vi "DevicesManager.vi"(8 "error in (no error)":errorcluster, 10 "Notifiers":T1, 11 "All Message Queue Cluster":T2) -> (0 "error out":errorcluster)   [LabVIEW 2017]
doc: "Ce VI a pour but de géré la connection des différents appareils.\n- Il permet de les connecté en fonction de leur port.\n- Il indique s'il se sont bien connecter et si tout se passe bien."
uses:
  Lib QMH/AllMessageQueue Cluster.ctl
  Lib QMH/Message Cluster.ctl
  Lib Notifier/Notifier.ctl
  Manager UI Data.ctl
  Lib QMH/MessageQueues.lvlib
  Lib Notifier/Notifier.lvlib
panel:
  in  "Portnumber Laser":i32(ring)=24 items=["COM1", "COM2", "COM3", "COM4", "COM5", "COM6", "COM7", "COM8", "COM9", "COM10", "COM11", "COM12", "COM13", "COM14", "COM15", "COM16", "COM17", "COM18", "COM19", "COM20", "COM21", "COM22", "COM23", "COM24", "COM25", "COM26", "COM27", "COM28", "COM29", "COM30"]
  out "Laser Initialized":bool
  out "Status Laser":string
  in  "Connect Laser":bool
  in  "Port Number Slit":i32(ring)=2 items=["COM1", "COM2", "COM3", "COM4", "COM5", "COM6", "COM7", "COM8", "COM9", "COM10", "COM11", "COM12", "COM13", "COM14", "COM15", "COM16", "COM17", "COM18", "COM19", "COM20", "COM21", "COM22", "COM23", "COM24", "COM25", "COM26", "COM27", "COM28", "COM29", "COM30"]
  in  "Portnumber Positioner":i32(ring)=17 items=["COM1", "COM2", "COM3", "COM4", "COM5", "COM6", "COM7", "COM8", "COM9", "COM10", "COM11", "COM12", "COM13", "COM14", "COM15", "COM16", "COM17", "COM18", "COM19", "COM20", "COM21", "COM22", "COM23", "COM24", "COM25", "COM26", "COM27", "COM28", "COM29", "COM30"]
  out "Positioner Initialized":bool
  out "Spectro Initialized":bool
  out "Slit Initialized":bool
  out "Status Spectro":string
  out "Status Slit":string
  out "Status Positioner":string
  in  "Connect Positioner":bool
  in  "Connect Slit":bool
  in  "Connect Spectro":bool
  # "Spectrometer"
  # "Slit"
  # "Selector"
  # "Laser"
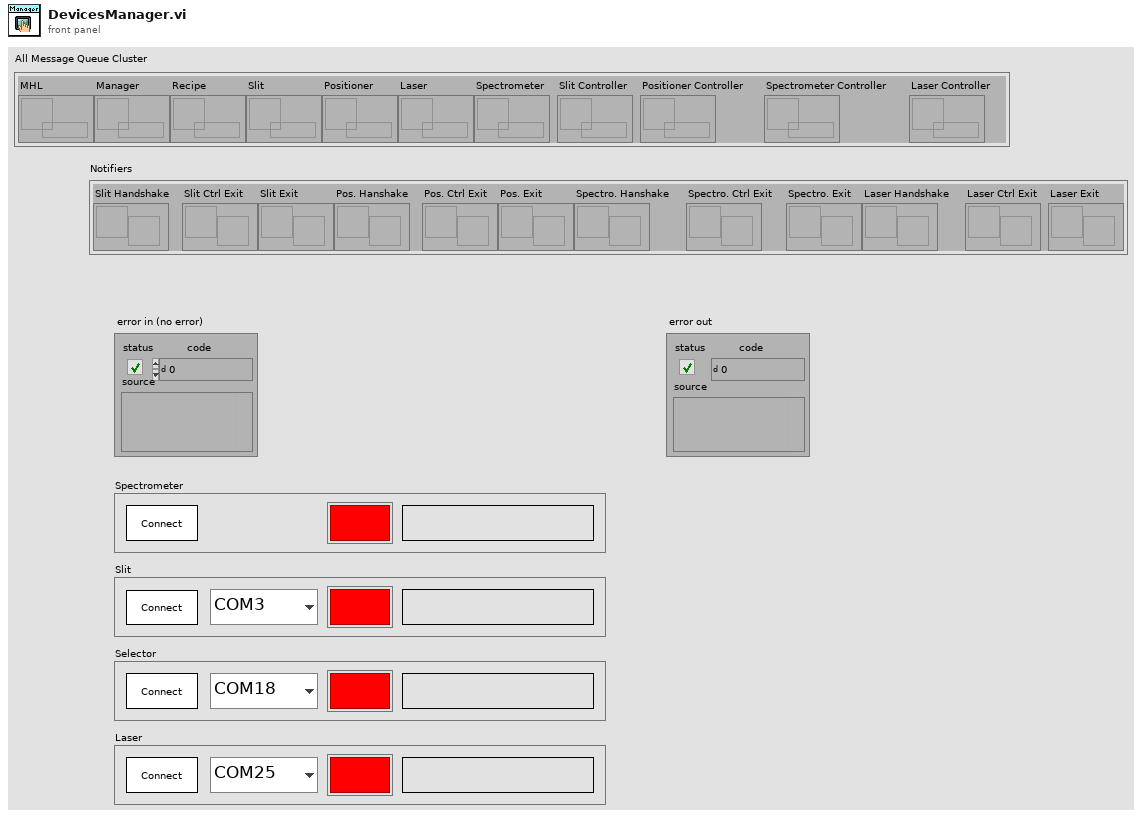
[diagram p1: front panel]
types:
  T1 = typedef "Notifier.lvlib/Notifier.ctl" = cluster{"Slit Handshake":refnum<notifier>, "Slit Ctrl Exit":refnum<notifier>, "Slit Exit":refnum<notifier>, "Pos. Hanshake":refnum<notifier>, "Pos. Ctrl Exit":refnum<notifier>, "Pos. Exit":refnum<notifier>, "Spectro. Hanshake":refnum<notifier>, "Spectro. Ctrl Exit":refnum<notifier>, "Spectro. Exit":refnum<notifier>, "Laser Handshake":refnum<notifier>, "Laser Ctrl Exit":refnum<notifier>, "Laser Exit":refnum<notifier>}
  T2 = typedef "MessageQueues.lvlib/AllMessageQueue Cluster.ctl" = cluster{"MHL":refnum<queue>, "Manager":refnum<queue>, "Recipe":refnum<queue>, "Slit":refnum<queue>, "Positioner":refnum<queue>, "Laser":refnum<queue>, "Spectrometer":refnum<queue>, "Slit Controller":refnum<queue>, "Positioner Controller":refnum<queue>, "Spectrometer Controller":refnum<queue>, "Laser Controller":refnum<queue>}
  T3 = typedef "Manager UI Data.ctl" = cluster{"Spectro Initialized":bool, "Status Spectro":string, "Slit Initialized":bool, "Status Slit":string, "Positioner Initialized":bool, "Status Positioner":string, "Laser Initialized":bool, "Status Laser":string}
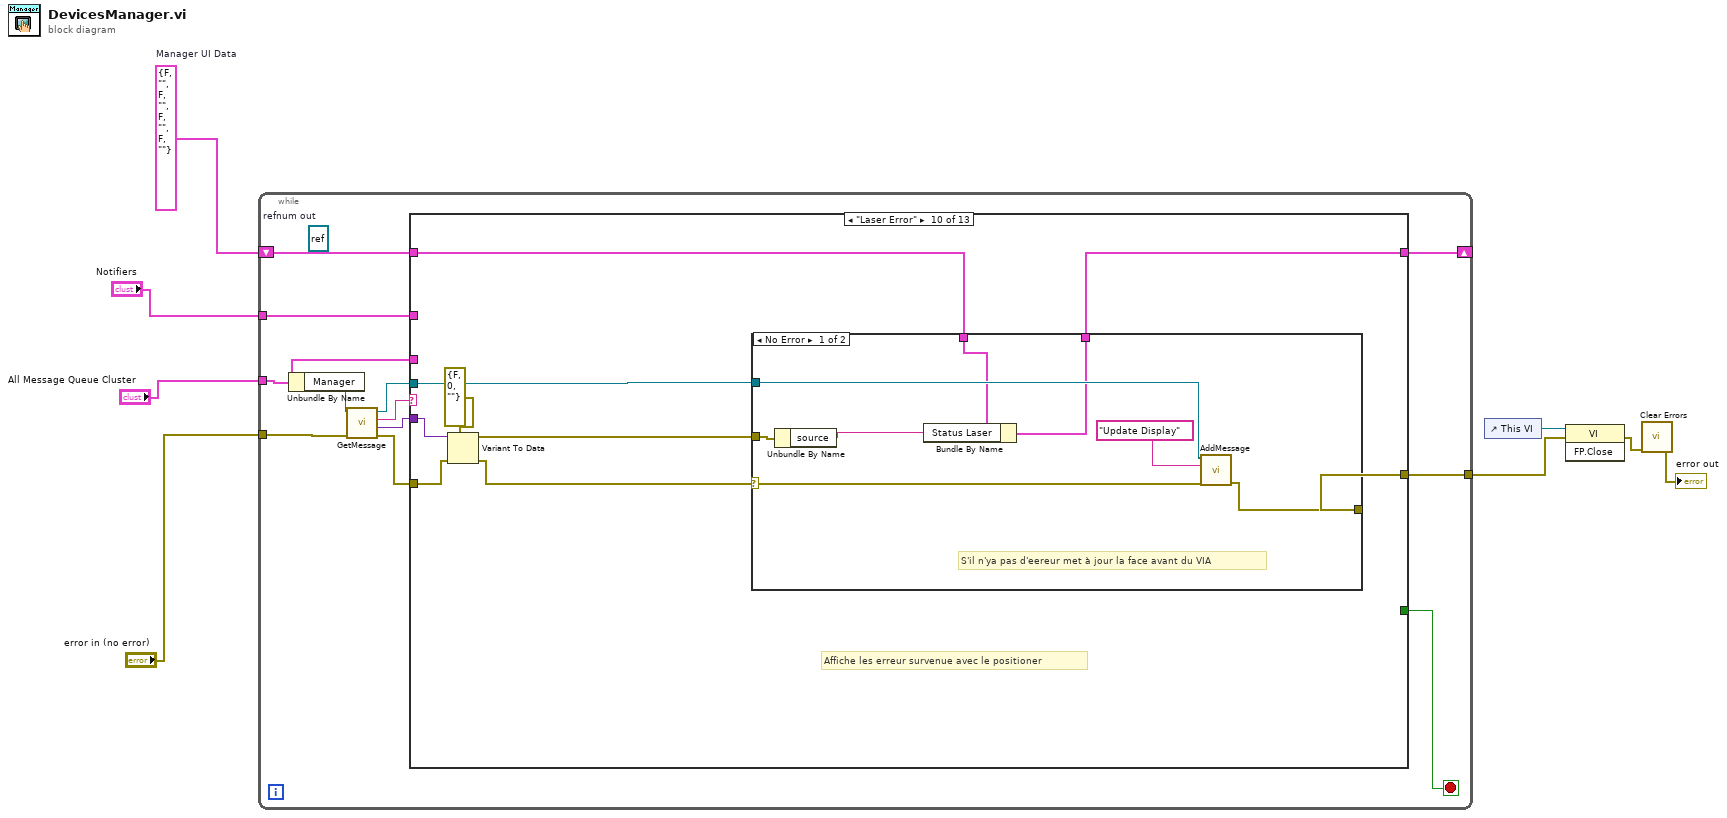
[diagram p0: block diagram]
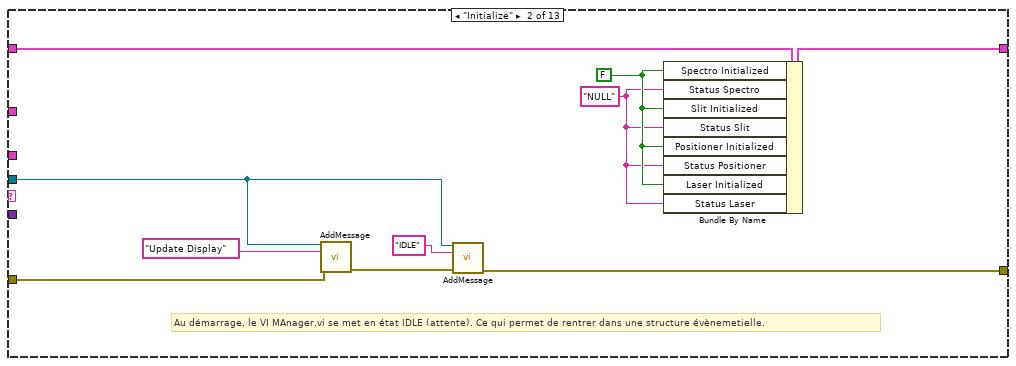
[diagram p3: hidden frame]
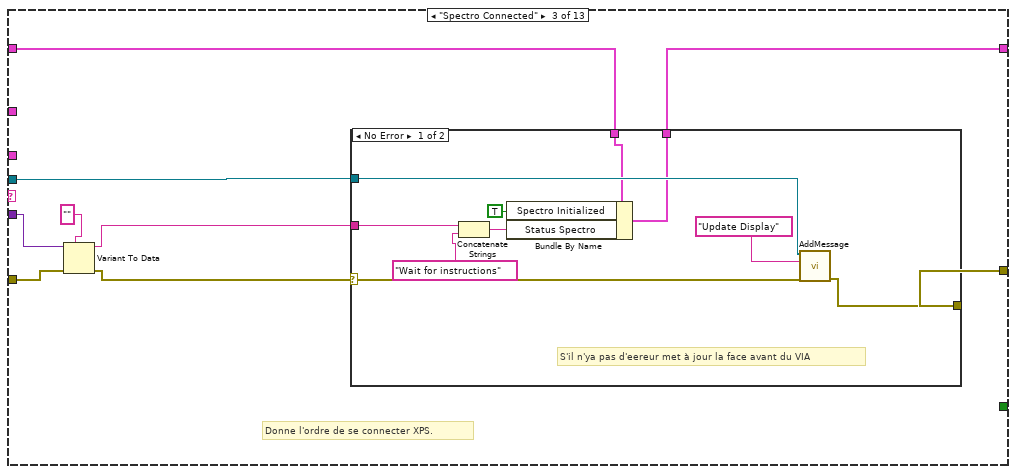
[diagram p4: hidden frame]
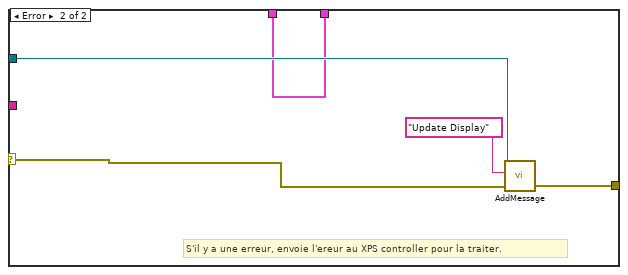
[diagram p5: hidden frame]
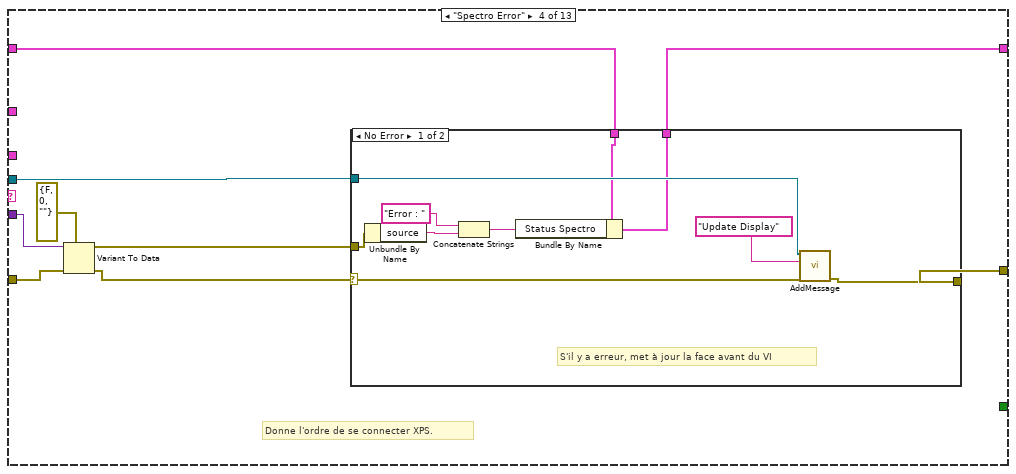
[diagram p6: hidden frame]
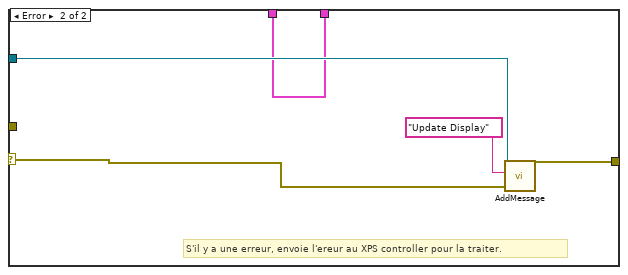
[diagram p7: hidden frame]
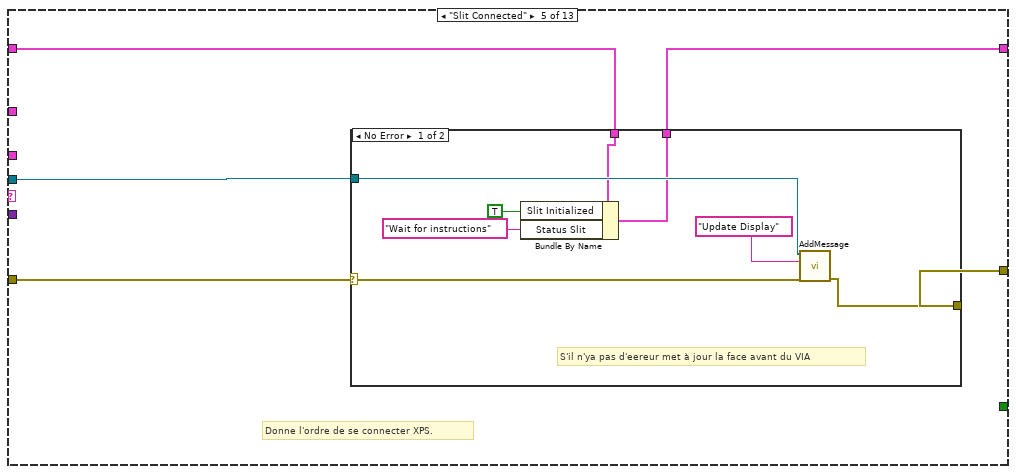
[diagram p8: hidden frame]
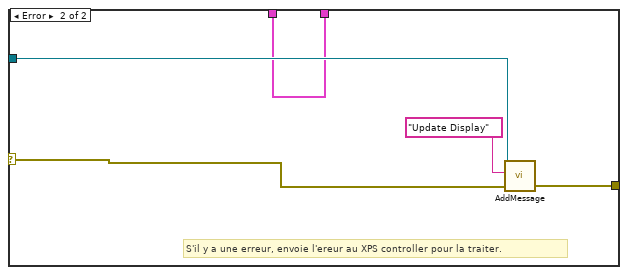
[diagram p9: hidden frame]
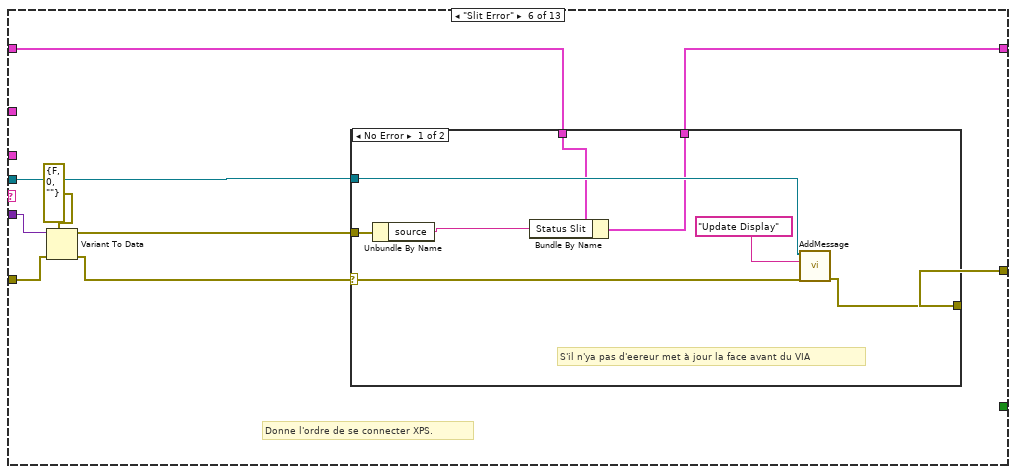
[diagram p10: hidden frame]
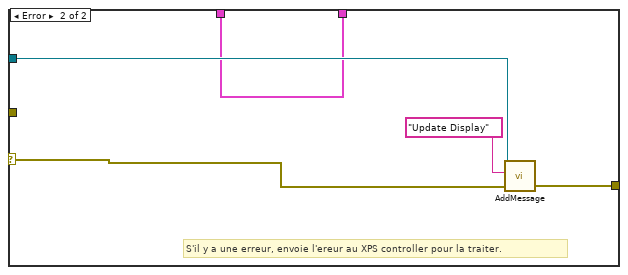
[diagram p11: hidden frame]
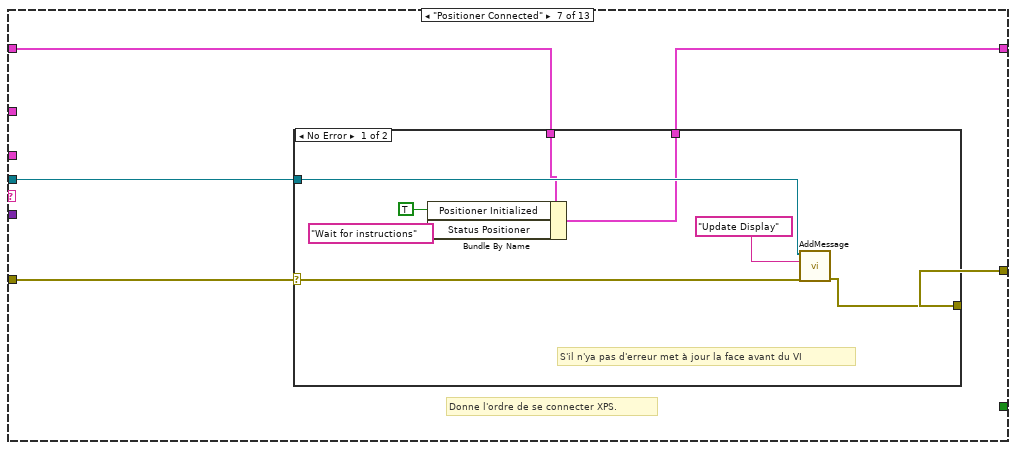
[diagram p12: hidden frame]
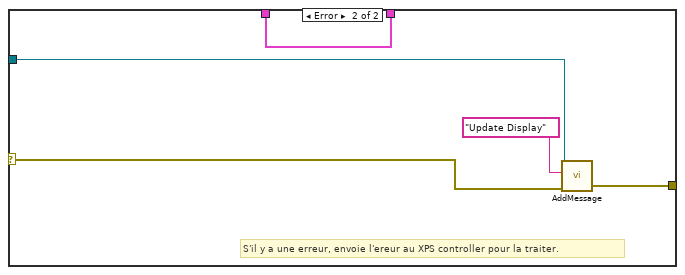
[diagram p13: hidden frame]
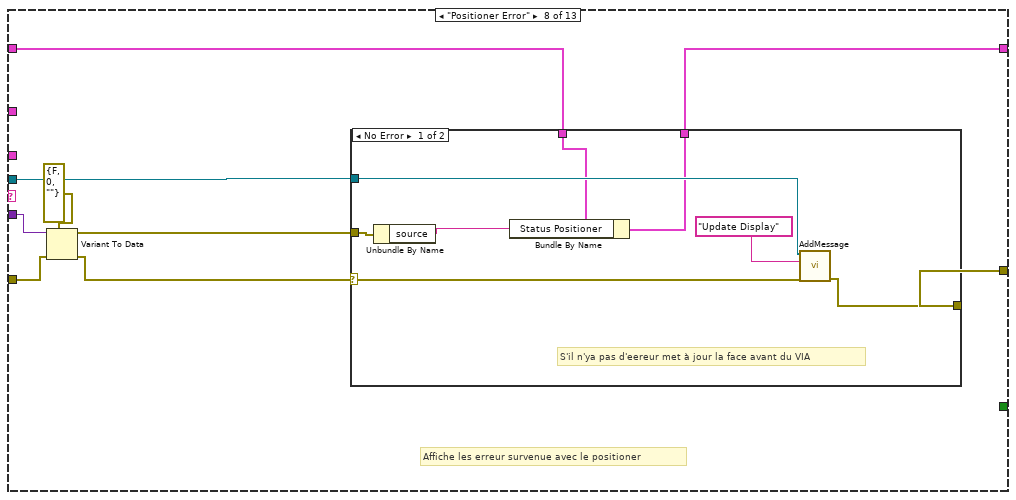
[diagram p14: hidden frame]
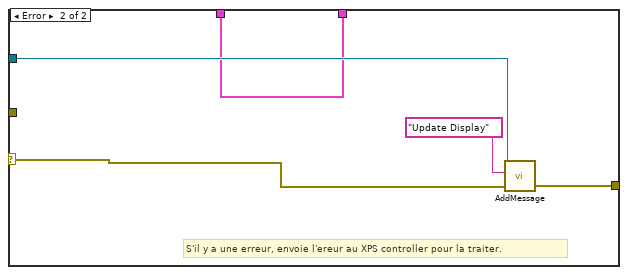
[diagram p15: hidden frame]
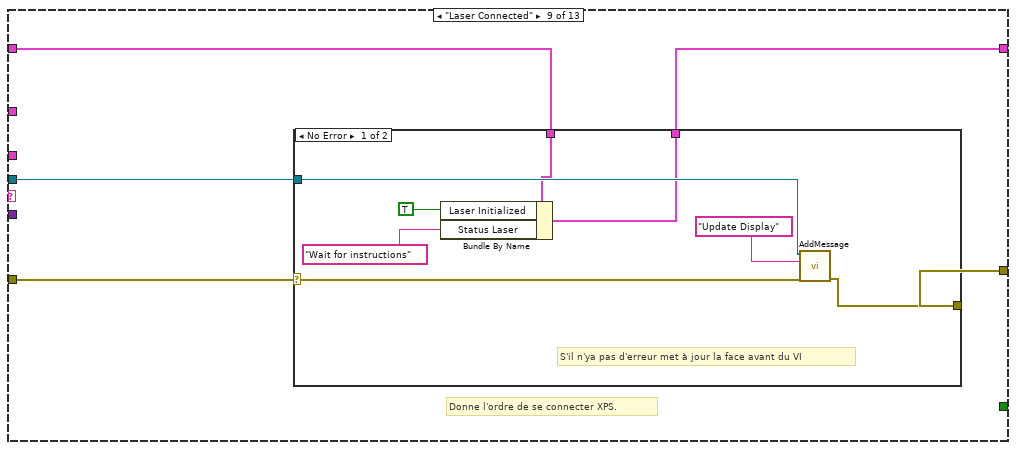
[diagram p16: hidden frame]
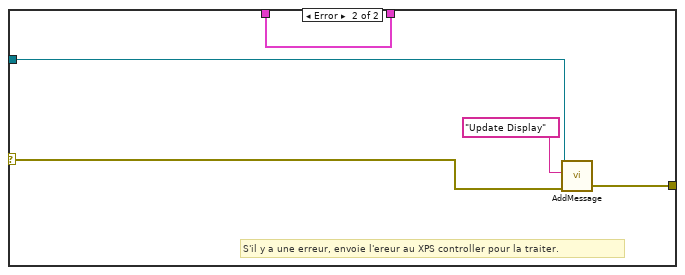
[diagram p17: hidden frame]
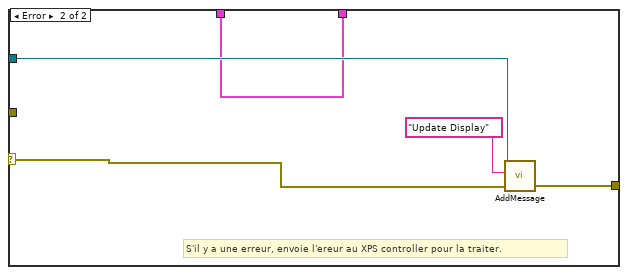
[diagram p18: hidden frame]
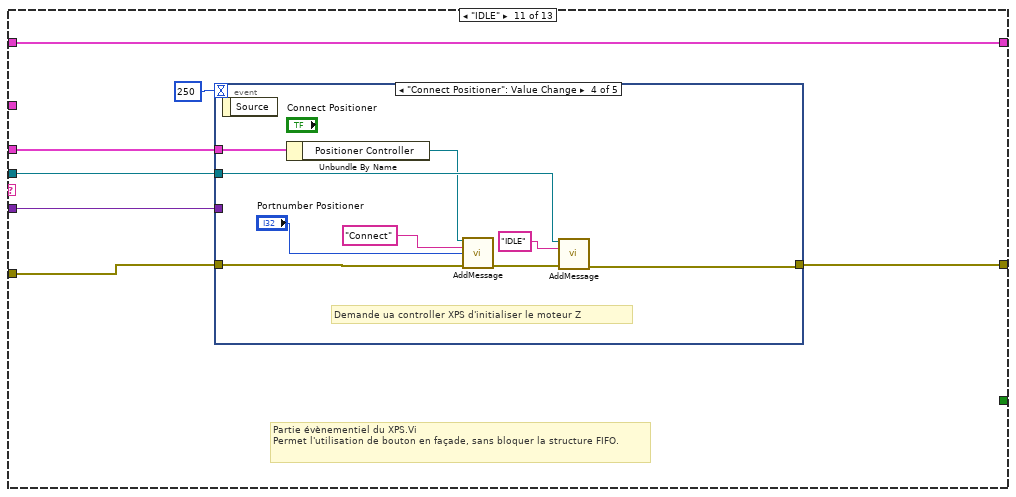
[diagram p19: hidden frame]
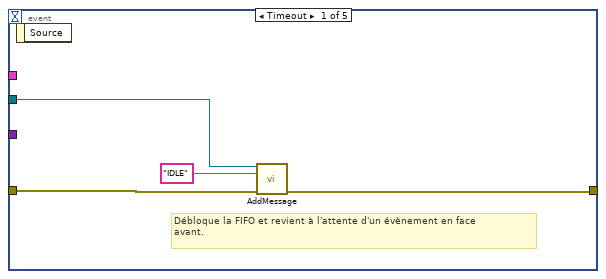
[diagram p20: hidden frame]
diagram:
  w5 = T3 {"Spectro Initialized"=FALSE, "Status Spectro"="", "Slit Initialized"=FALSE, "Status Slit"="", "Positioner Initialized"=FALSE, "Status Positioner"="", "Laser Initialized"=FALSE, "Status Laser"=""}  # Manager UI Data
  (unwired) refnum<file> refnum  # refnum out
  n1 = while {
    tunnel: "All Message Queue Cluster" -> [w9]
    tunnel: "Notifiers" -> [w20]
    tunnel: "error in (no error)" -> [w14]
    tunnel: [w13] -> w2
    shift-right: [w10] -> _
    shift-left: w5 -> [w11]
    stop <- w12 stop-if-true
    n2 = Unbundle By Name(w9) -> ("Manager"=w19:refnum<queue>)
    n3 = call "GetMessage.vi"("entrée d'erreur"=w14, "Message queue"=w19) -> ("sortie d'erreur"=w15:errorcluster, "Data"=w16:variant, "Message"=w17:string, "Dup Message Queue"=w18:refnum<queue>)  [unwired: 6 in]
    n4 = case shown="\"Laser Error\"" w17 {
      tunnel: w20 -> [_ _ _ _ _ _ _ _ _ _ _ _ _]
      tunnel: w18 -> [_ w26 w41 w65 w85 w107 w125 w147 w165 w187 w206 _ w259]
      tunnel: w16 -> [_ _ w35 w59 _ w101 _ w141 _ w181 w205 _ _]
      tunnel: w15 -> [w22 w28 w37 w61 w81 w103 w121 w143 w161 w183 w204 w256 w260]
      tunnel: [w22 w31 w40 w64 w84 w106 w124 w146 w164 w186 w203 w256 w257] -> w13
      tunnel: [_ _ _ _ _ _ _ _ _ _ _ _ TRUE] -> w12
      tunnel: w11 -> [w21 w30 w39 w63 w83 w105 w123 w145 w163 w185 w202 w255 w258]
      tunnel: [w21 w29 w38 w62 w82 w104 w122 w144 w162 w184 w202 w255 w258] -> w10
      tunnel: w9 -> [_ _ _ _ _ _ _ _ _ _ w201 _ _]
      frame Default {
        # "ne fait rien si le message dépilé n'existe pas"
      }
      frame "Initialize" {
        w23 = "NULL" ("Status Spectro")
        w24 = FALSE ("Spectro Initialized")
        # "Au démarrage, le VI MAnager.vi se met en état IDLE (attente). Ce qui permet de rentrer dans une structure évènemetielle."
        n5 = call "AddMessage.vi"("Message queue"=w26, "Message"="Update Display", "entrée d'erreur (pas d'erreur)"=w28) -> ("error out"=w27:errorcluster)  [unwired: 11 in, 1 out]
        n6 = call "AddMessage.vi"("Message queue"=w26, "Message"="IDLE", "entrée d'erreur (pas d'erreur)"=w27) -> ("error out"=w31:errorcluster)  [unwired: 11 in, 1 out]
        n7 = Bundle By Name(cluster=w30, "Spectro Initialized"=w24, "Status Spectro"=w23, "Slit Initialized"=w24, "Status Slit"=w23, "Positioner Initialized"=w24, "Status Positioner"=w23, "Laser Initialized"=w24, "Status Laser"=w23) -> (w29:T3)
      }
      frame "Spectro Connected" {
        # "Donne l'ordre de se connecter XPS."
        n8 = Variant To Data(error in=w37, type="", Variant=w35) -> (data=w33:string, error out=w36:errorcluster)
        n9 = case shown="No Error" w36 {
          selector: w36 -> [w49 w52]
          tunnel: w41 -> [w51 w56]
          tunnel: [w48 w54] -> w40
          tunnel: w39 -> [w47 w53]
          tunnel: [w46 w53] -> w38
          tunnel: w33 -> [w42 _]
          frame No Error {
            # "S'il n'ya pas d'eereur met à jour la face avant du VIA"
            n10 = Concatenate Strings(w42, "Wait for instructions" ("Status Spectro")) -> (w43:string)
            n11 = Bundle By Name(cluster=w47, "Spectro Initialized"=TRUE, "Status Spectro"=w43) -> (w46:T3)
            n12 = call "AddMessage.vi"("Message queue"=w51, "Message"="Update Display", "entrée d'erreur (pas d'erreur)"=w49) -> ("error out"=w48:errorcluster)  [unwired: 11 in, 1 out]
          }
          frame Error {
            # "S'il y a une erreur, envoie l'ereur au XPS controller pour la traiter."
            n13 = call "AddMessage.vi"("Message queue"=w56, "Message"="Update Display", "entrée d'erreur (pas d'erreur)"=w52) -> ("error out"=w54:errorcluster)  [unwired: 11 in, 1 out]
          }
        }
      }
      frame "Spectro Error" {
        # "Donne l'ordre de se connecter XPS."
        n14 = Variant To Data(error in=w61, type=errorcluster {"status"=FALSE, "code"=0, "source"=""} ("error out"), Variant=w59) -> (data=w57:errorcluster, error out=w60:errorcluster)
        n15 = case shown="No Error" w60 {
          selector: w60 -> [w73 w76]
          tunnel: w65 -> [w75 w80]
          tunnel: [w72 w78] -> w64
          tunnel: w63 -> [w71 w77]
          tunnel: [w70 w77] -> w62
          tunnel: w57 -> [w68 _]
          frame No Error {
            # "S'il y a erreur, met à jour la face avant du VI"
            n16 = Unbundle By Name(w68) -> ("source"=w67:string)
            n17 = Concatenate Strings("Error : " ("string"), w67) -> (w69:string)
            n18 = Bundle By Name(cluster=w71, "Status Spectro"=w69) -> (w70:T3)
            n19 = call "AddMessage.vi"("Message queue"=w75, "Message"="Update Display", "entrée d'erreur (pas d'erreur)"=w73) -> ("error out"=w72:errorcluster)  [unwired: 11 in, 1 out]
          }
          frame Error {
            # "S'il y a une erreur, envoie l'ereur au XPS controller pour la traiter."
            n20 = call "AddMessage.vi"("Message queue"=w80, "Message"="Update Display", "entrée d'erreur (pas d'erreur)"=w76) -> ("error out"=w78:errorcluster)  [unwired: 11 in, 1 out]
          }
        }
      }
      frame "Slit Connected" {
        # "Donne l'ordre de se connecter XPS."
        n21 = case shown="No Error" w81 {
          selector: w81 -> [w91 w94]
          tunnel: w85 -> [w93 w98]
          tunnel: [w90 w96] -> w84
          tunnel: w83 -> [w89 w95]
          tunnel: [w88 w95] -> w82
          frame No Error {
            # "S'il n'ya pas d'eereur met à jour la face avant du VIA"
            n22 = Bundle By Name(cluster=w89, "Slit Initialized"=TRUE ("Spectro Initialized"), "Status Slit"="Wait for instructions" ("Status Spectro")) -> (w88:T3)
            n23 = call "AddMessage.vi"("Message queue"=w93, "Message"="Update Display", "entrée d'erreur (pas d'erreur)"=w91) -> ("error out"=w90:errorcluster)  [unwired: 11 in, 1 out]
          }
          frame Error {
            # "S'il y a une erreur, envoie l'ereur au XPS controller pour la traiter."
            n24 = call "AddMessage.vi"("Message queue"=w98, "Message"="Update Display", "entrée d'erreur (pas d'erreur)"=w94) -> ("error out"=w96:errorcluster)  [unwired: 11 in, 1 out]
          }
        }
      }
      frame "Slit Error" {
        # "Donne l'ordre de se connecter XPS."
        n25 = Variant To Data(error in=w103, type=errorcluster {"status"=FALSE, "code"=0, "source"=""} ("error out"), Variant=w101) -> (data=w99:errorcluster, error out=w102:errorcluster)
        n26 = case shown="No Error" w102 {
          selector: w102 -> [w113 w116]
          tunnel: w107 -> [w115 w120]
          tunnel: [w112 w118] -> w106
          tunnel: w105 -> [w111 w117]
          tunnel: [w110 w117] -> w104
          tunnel: w99 -> [w109 _]
          frame No Error {
            # "S'il n'ya pas d'eereur met à jour la face avant du VIA"
            n27 = Unbundle By Name(w109) -> ("source"=w108:string)
            n28 = Bundle By Name(cluster=w111, "Status Slit"=w108) -> (w110:T3)
            n29 = call "AddMessage.vi"("Message queue"=w115, "Message"="Update Display", "entrée d'erreur (pas d'erreur)"=w113) -> ("error out"=w112:errorcluster)  [unwired: 11 in, 1 out]
          }
          frame Error {
            # "S'il y a une erreur, envoie l'ereur au XPS controller pour la traiter."
            n30 = call "AddMessage.vi"("Message queue"=w120, "Message"="Update Display", "entrée d'erreur (pas d'erreur)"=w116) -> ("error out"=w118:errorcluster)  [unwired: 11 in, 1 out]
          }
        }
      }
      frame "Positioner Connected" {
        # "Donne l'ordre de se connecter XPS."
        n31 = case shown="No Error" w121 {
          selector: w121 -> [w131 w134]
          tunnel: w125 -> [w133 w138]
          tunnel: [w130 w136] -> w124
          tunnel: w123 -> [w129 w135]
          tunnel: [w128 w135] -> w122
          frame No Error {
            # "S'il n'ya pas d'erreur met à jour la face avant du VI"
            n32 = Bundle By Name(cluster=w129, "Positioner Initialized"=TRUE ("Spectro Initialized"), "Status Positioner"="Wait for instructions" ("Status Spectro")) -> (w128:T3)
            n33 = call "AddMessage.vi"("Message queue"=w133, "Message"="Update Display", "entrée d'erreur (pas d'erreur)"=w131) -> ("error out"=w130:errorcluster)  [unwired: 11 in, 1 out]
          }
          frame Error {
            # "S'il y a une erreur, envoie l'ereur au XPS controller pour la traiter."
            n34 = call "AddMessage.vi"("Message queue"=w138, "Message"="Update Display", "entrée d'erreur (pas d'erreur)"=w134) -> ("error out"=w136:errorcluster)  [unwired: 11 in, 1 out]
          }
        }
      }
      frame "Positioner Error" {
        # "Affiche les erreur survenue avec le positioner"
        n35 = Variant To Data(error in=w143, type=errorcluster {"status"=FALSE, "code"=0, "source"=""} ("error out"), Variant=w141) -> (data=w139:errorcluster, error out=w142:errorcluster)
        n36 = case shown="No Error" w142 {
          selector: w142 -> [w153 w156]
          tunnel: w147 -> [w155 w160]
          tunnel: [w152 w158] -> w146
          tunnel: w145 -> [w151 w157]
          tunnel: [w150 w157] -> w144
          tunnel: w139 -> [w149 _]
          frame No Error {
            # "S'il n'ya pas d'eereur met à jour la face avant du VIA"
            n37 = Unbundle By Name(w149) -> ("source"=w148:string)
            n38 = Bundle By Name(cluster=w151, "Status Positioner"=w148) -> (w150:T3)
            n39 = call "AddMessage.vi"("Message queue"=w155, "Message"="Update Display", "entrée d'erreur (pas d'erreur)"=w153) -> ("error out"=w152:errorcluster)  [unwired: 11 in, 1 out]
          }
          frame Error {
            # "S'il y a une erreur, envoie l'ereur au XPS controller pour la traiter."
            n40 = call "AddMessage.vi"("Message queue"=w160, "Message"="Update Display", "entrée d'erreur (pas d'erreur)"=w156) -> ("error out"=w158:errorcluster)  [unwired: 11 in, 1 out]
          }
        }
      }
      frame "Laser Connected" {
        # "Donne l'ordre de se connecter XPS."
        n41 = case shown="No Error" w161 {
          selector: w161 -> [w171 w174]
          tunnel: w165 -> [w173 w178]
          tunnel: [w170 w176] -> w164
          tunnel: w163 -> [w169 w175]
          tunnel: [w168 w175] -> w162
          frame No Error {
            # "S'il n'ya pas d'erreur met à jour la face avant du VI"
            n42 = Bundle By Name(cluster=w169, "Laser Initialized"=TRUE ("Spectro Initialized"), "Status Laser"="Wait for instructions" ("Status Spectro")) -> (w168:T3)
            n43 = call "AddMessage.vi"("Message queue"=w173, "Message"="Update Display", "entrée d'erreur (pas d'erreur)"=w171) -> ("error out"=w170:errorcluster)  [unwired: 11 in, 1 out]
          }
          frame Error {
            # "S'il y a une erreur, envoie l'ereur au XPS controller pour la traiter."
            n44 = call "AddMessage.vi"("Message queue"=w178, "Message"="Update Display", "entrée d'erreur (pas d'erreur)"=w174) -> ("error out"=w176:errorcluster)  [unwired: 11 in, 1 out]
          }
        }
      }
      frame "Laser Error" {
        # "Affiche les erreur survenue avec le positioner"
        n45 = Variant To Data(error in=w183, type=errorcluster {"status"=FALSE, "code"=0, "source"=""} ("error out"), Variant=w181) -> (data=w179:errorcluster, error out=w182:errorcluster)
        n46 = case shown="No Error" w182 {
          selector: w182 -> [w193 w196]
          tunnel: w187 -> [w195 w200]
          tunnel: [w192 w198] -> w186
          tunnel: w185 -> [w191 w197]
          tunnel: [w190 w197] -> w184
          tunnel: w179 -> [w189 _]
          frame No Error {
            # "S'il n'ya pas d'eereur met à jour la face avant du VIA"
            n47 = Unbundle By Name(w189) -> ("source"=w188:string)
            n48 = Bundle By Name(cluster=w191, "Status Laser"=w188) -> (w190:T3)
            n49 = call "AddMessage.vi"("Message queue"=w195, "Message"="Update Display", "entrée d'erreur (pas d'erreur)"=w193) -> ("error out"=w192:errorcluster)  [unwired: 11 in, 1 out]
          }
          frame Error {
            # "S'il y a une erreur, envoie l'ereur au XPS controller pour la traiter."
            n50 = call "AddMessage.vi"("Message queue"=w200, "Message"="Update Display", "entrée d'erreur (pas d'erreur)"=w196) -> ("error out"=w198:errorcluster)  [unwired: 11 in, 1 out]
          }
        }
      }
      frame "IDLE" {
        # "Partie évènementiel du XPS.Vi\nPermet l'utilisation de bouton en façade, sans bloquer la structure FIFO."
        n51 = event shown="[3] \"Connect Positioner\": Value Change" {
          selector: _ -> [_ _ _ _ _]
          dyn-events: _ -> [_ _ _ _ _]
          timeout: 250 -> [_ _ _ _ _]
          tunnel: w206 -> [w211 w214 w223 w232 w241]
          tunnel: w205 -> [_ _ _ _ _]
          tunnel: w204 -> [w210 w219 w228 w237 w246]
          tunnel: [w209 w216 w225 w234 w243] -> w203
          tunnel: w201 -> [_ w213 w222 w231 w240]
          event Timeout {
            # "Débloque la FIFO et revient à l'attente d'un évènement en face\navant."
            n52 = event-data() -> ()  [unwired: 1 in, 1 out]
            n53 = call "AddMessage.vi"("Message queue"=w211, "Message"="IDLE", "entrée d'erreur (pas d'erreur)"=w210) -> ("error out"=w209:errorcluster)  [unwired: 11 in, 1 out]
          }
          event "Connect Spectro": Value Change {
            # "Demande au controller d'initialiser le moteur X"
            n54 = event-data() -> ()  [unwired: 1 in, 1 out]
            n55 = Unbundle By Name(w213) -> ("Spectrometer Controller"=w212:refnum<queue>)
            n56 = call "AddMessage.vi"("Message queue"=w212, "Message"="Connect", "entrée d'erreur (pas d'erreur)"=w219) -> ("error out"=w217:errorcluster)  [unwired: 11 in, 1 out]
            n57 = call "AddMessage.vi"("Message queue"=w214, "Message"="IDLE", "entrée d'erreur (pas d'erreur)"=w217) -> ("error out"=w216:errorcluster)  [unwired: 11 in, 1 out]
          }
          event "Connect Slit": Value Change {
            # "Demande au controller XPS d'initialiser le moteur Y"
            n58 = event-data() -> ()  [unwired: 1 in, 1 out]
            n59 = Unbundle By Name(w222) -> ("Slit Controller"=w221:refnum<queue>)
            n60 = call "AddMessage.vi"("Message queue"=w221, "Message"="Connect", "Data"="Port Number Slit", "entrée d'erreur (pas d'erreur)"=w228) -> ("error out"=w226:errorcluster)  [unwired: 10 in, 1 out]
            n61 = call "AddMessage.vi"("Message queue"=w223, "Message"="IDLE", "entrée d'erreur (pas d'erreur)"=w226) -> ("error out"=w225:errorcluster)  [unwired: 11 in, 1 out]
          }
          event "Connect Positioner": Value Change {
            # "Demande ua controller XPS d'initialiser le moteur Z"
            n62 = event-data() -> ()  [unwired: 1 in, 1 out]
            n63 = Unbundle By Name(w231) -> ("Positioner Controller"=w230:refnum<queue>)
            n64 = call "AddMessage.vi"("Message queue"=w230, "Message"="Connect", "Data"="Portnumber Positioner", "entrée d'erreur (pas d'erreur)"=w237) -> ("error out"=w235:errorcluster)  [unwired: 10 in, 1 out]
            n65 = call "AddMessage.vi"("Message queue"=w232, "Message"="IDLE", "entrée d'erreur (pas d'erreur)"=w235) -> ("error out"=w234:errorcluster)  [unwired: 11 in, 1 out]
          }
          event "Connect Laser": Value Change {
            # "Demande ua controller XPS d'initialiser le moteur Z"
            n66 = event-data() -> ()  [unwired: 1 in, 1 out]
            n67 = Unbundle By Name(w240) -> ("Laser Controller"=w239:refnum<queue>)
            n68 = call "AddMessage.vi"("Message queue"=w239, "Message"="Connect", "Data"="Portnumber Laser", "entrée d'erreur (pas d'erreur)"=w246) -> ("error out"=w244:errorcluster)  [unwired: 10 in, 1 out]
            n69 = call "AddMessage.vi"("Message queue"=w241, "Message"="IDLE", "entrée d'erreur (pas d'erreur)"=w244) -> ("error out"=w243:errorcluster)  [unwired: 11 in, 1 out]
          }
        }
      }
      frame "Update Display" {
        # "Met à jour les valeur de status"
        n70 = Unbundle By Name(w255) -> ("Spectro Initialized"=→"Spectro Initialized":bool, "Status Spectro"=→"Status Spectro":string, "Slit Initialized"=→"Slit Initialized":bool, "Status Slit"=→"Status Slit":string, "Positioner Initialized"=→"Positioner Initialized":bool, "Status Positioner"=→"Status Positioner":string, "Laser Initialized"=→"Laser Initialized":bool, "Status Laser"=→"Status Laser":string)
      }
      frame "Exit" {
        n71 = Release Queue(queue=w259, error in (no error)=w260) -> (error out=w257:errorcluster)  [unwired: 1 in, 2 out]
      }
    }
  }
  n72 = control-ref of="This VI"() -> (w4:refnum<vi>)
  n73 = invoke class="VI" method="FP.Close"(reference=w4, error in=w2) -> (error out=w3:errorcluster)  [unwired: 1 in, 2 out]
  n74 = call <vilib>:"Clear Errors.vi"("error in (no error)"=w3) -> ("error out"=→"error out":errorcluster)  [unwired: 5 in, 1 out]
